vi "tm484_DSP.vi"() -> ()   [LabVIEW 2011]
panel:
  in  "SC Enable":bool
  in  "BG Enable":bool
  in  "Frame Averaging":i32(ring)=1 items=["1 Frame"=1, "2 Frames"=2, "4 Frames"=4]
  in  "Recursive Frames":i32(ring)=1 items=["1 Frame"=1, "2 Frames"=2, "4 Frames"=4, "8 Frames"=8, "16 Frames"=16]
  out "Image":u16[][](graph)
  in  "Quit":bool
  out "Error Out":errorcluster {"code" format="%.0x"}
  # "This is an example how to use the DSP functions.\nNot all camera have the DSP functions. Please\ncheck your camera manual to see your camera's\ncapabilities."
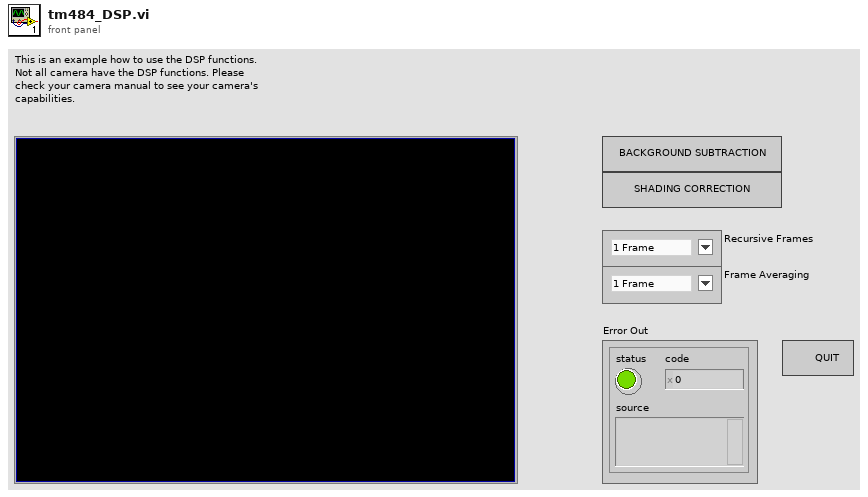
[diagram p1: front panel]
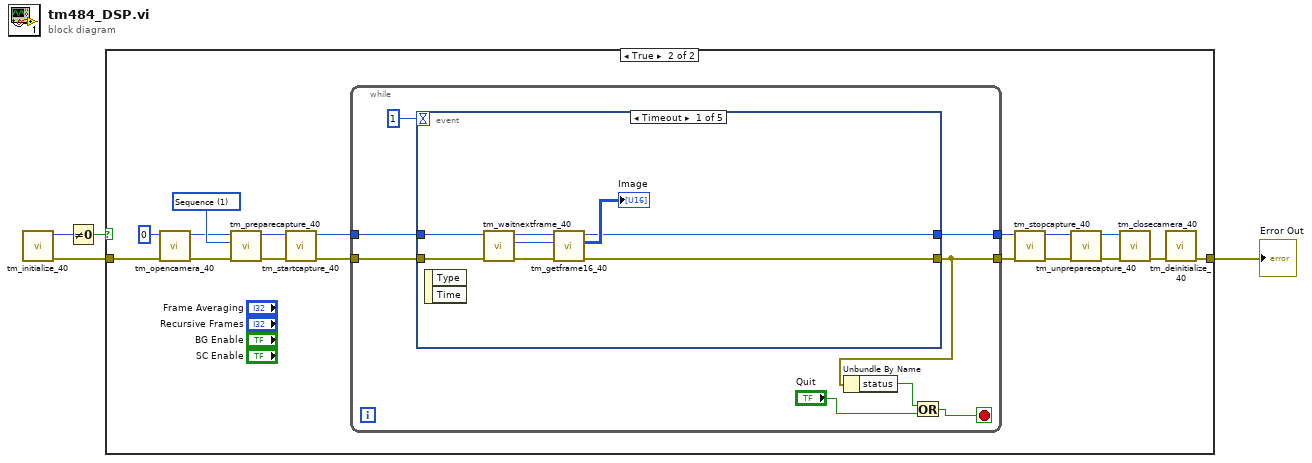
[diagram p0: block diagram]
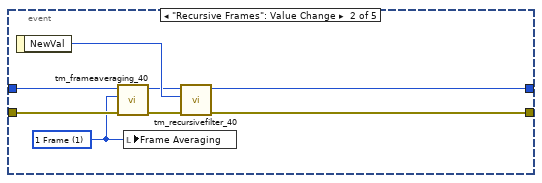
[diagram p3: hidden frame]
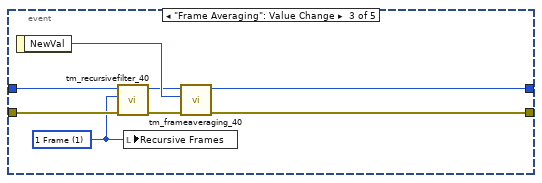
[diagram p4: hidden frame]
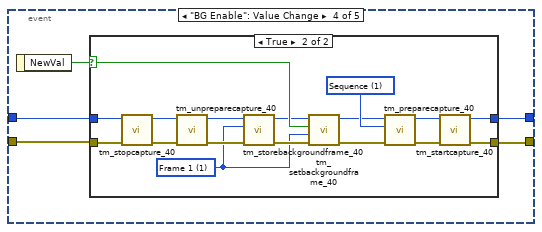
[diagram p5: hidden frame]
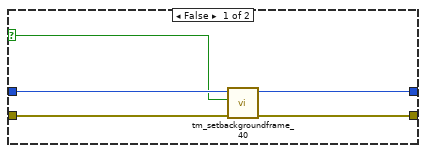
[diagram p6: hidden frame]
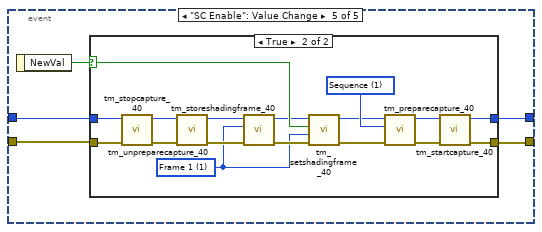
[diagram p7: hidden frame]
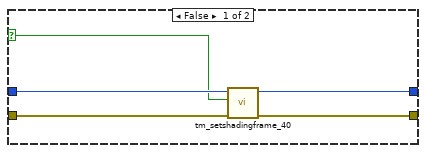
[diagram p8: hidden frame]
diagram:
  n1 = call <userlib>:"tm_initialize_40.vi"() -> ("error out"=w1:errorcluster, "Number Of Cameras"=w2:u32)  [unwired: 8 in, 2 out]
  n2 = Not Equal To 0?(x=w2) -> (x != 0?=w4:bool)
  n3 = case shown="True" w4 {
    tunnel: w1 -> [w5 w22]
    tunnel: [w5 w19] -> w3
    frame False {
    }
    frame True {
      w12 = 1 items=["Snap", "Sequence"] ("Capture mode")
      n4 = call <userlib>:"tm_opencamera_40.vi"("error in (no error)"=w22, "Camera Index"=u32 0) -> ("error out"=w9:errorcluster, "Handle out"=w8:u32)  [unwired: 7 in, 1 out]
      n5 = call <userlib>:"tm_preparecapture_40.vi"("error in (no error)"=w9, "Capture mode"=w12, "Handle in"=w8) -> ("error out"=w10:errorcluster, "Handle out"=w11:u32)  [unwired: 5 in, 2 out]
      n6 = call <userlib>:"tm_startcapture_40.vi"("error in (no error)"=w10, "Handle in"=w11) -> ("error out"=w6:errorcluster, "Handle out"=w7:u32)  [unwired: 8 in]
      n7 = while {
        tunnel: [w28] -> w15
        tunnel: [w24] -> w16
        tunnel: w7 -> [w30]
        tunnel: w6 -> [w29]
        stop <- w23 stop-if-true
        n8 = event shown="[0] Timeout" {
          selector: _ -> [_ _ _ _ _]
          dyn-events: _ -> [_ _ _ _ _]
          timeout: 1 -> [_ _ _ _ _]
          tunnel: w30 -> [w34 w42 w50 w58 w85]
          tunnel: w29 -> [w33 w43 w51 w57 w84]
          tunnel: [w31 w45 w53 w56 w83] -> w28
          tunnel: [w32 w44 w52 w55 w82] -> w24
          event Timeout {
            n9 = event-data() -> ()  [unwired: 1 in, 2 out]
            n10 = call <userlib>:"tm_waitnextframe_40.vi"("error in (no error)"=w33, "Handle in"=w34) -> ("error out"=w36:errorcluster, "Frame Index"=w38:i32, "Handle out"=w35:u32)  [unwired: 6 in, 1 out]
            n11 = call <userlib>:"tm_getframe16_40.vi"("error in (no error)"=w36, "Frame Index"=w38, "Handle in"=w35) -> ("error out"=w32:errorcluster, "Data"=→"Image":u16[][], "Handle out"=w31:u32)  [unwired: 5 in, 1 out]
          }
          event "Recursive Frames": Value Change {
            w39 = 1 items=["1 Frame"=1, "2 Frames"=2, "4 Frames"=4, "8 Frames"=8, "16 Frames"=16] ("Frames")
            n12 = event-data() -> ("NewVal"=w46:i32)  [unwired: 1 in]
            n13 = call <userlib>:"tm_frameaveraging_40.vi"("error in (no error)"=w43, "Frames"=w39, "Handle in"=w42) -> ("error out"=w40:errorcluster, "Handle out"=w41:u32)  [unwired: 7 in]
            n14 = local write "Frame Averaging"(w39) -> ()
            n15 = call <userlib>:"tm_recursivefilter_40.vi"("error in (no error)"=w40, "Frames"=w46, "Handle in"=w41) -> ("error out"=w44:errorcluster, "Handle out"=w45:u32)  [unwired: 7 in]
          }
          event "Frame Averaging": Value Change {
            w47 = 1 items=["1 Frame"=1, "2 Frames"=2, "4 Frames"=4, "8 Frames"=8, "16 Frames"=16] ("Frames")
            n16 = event-data() -> ("NewVal"=w54:i32)  [unwired: 1 in]
            n17 = call <userlib>:"tm_recursivefilter_40.vi"("error in (no error)"=w51, "Frames"=w47, "Handle in"=w50) -> ("error out"=w48:errorcluster, "Handle out"=w49:u32)  [unwired: 7 in]
            n18 = local write "Recursive Frames"(w47) -> ()
            n19 = call <userlib>:"tm_frameaveraging_40.vi"("error in (no error)"=w48, "Frames"=w54, "Handle in"=w49) -> ("error out"=w52:errorcluster, "Handle out"=w53:u32)  [unwired: 7 in]
          }
          event "BG Enable": Value Change {
            n20 = event-data() -> ("NewVal"=w59:bool)  [unwired: 1 in]
            n21 = case shown="True" w59 {
              selector: w59 -> [w60 w75]
              tunnel: w58 -> [w64 w78]
              tunnel: w57 -> [w63 w79]
              tunnel: [w62 w66] -> w56
              tunnel: [w61 w65] -> w55
              frame False {
                n22 = call <userlib>:"tm_setbackgroundframe_40.vi"("error in (no error)"=w63, "Enable"=w60, "Handle in"=w64) -> ("error out"=w61:errorcluster, "Handle out"=w62:u32)  [unwired: 7 in]
              }
              frame True {
                w69 = 1 items=["Snap", "Sequence"] ("Capture mode")
                w72 = 1 items=["Frame 1"=1, "Frame 2"=2, "Frame 3"=3, "Frame 4"=4] ("Frame")
                n23 = call <userlib>:"tm_stopcapture_40.vi"("error in (no error)"=w79, "Handle in"=w78) -> ("error out"=w81:errorcluster, "Handle out"=w80:u32)  [unwired: 8 in]
                n24 = call <userlib>:"tm_unpreparecapture_40.vi"("error in (no error)"=w81, "Handle in"=w80) -> ("error out"=w76:errorcluster, "Handle out"=w77:u32)  [unwired: 8 in]
                n25 = call <userlib>:"tm_storebackgroundframe_40.vi"("error in (no error)"=w76, "Frame"=w72, "Handle in"=w77) -> ("error out"=w73:errorcluster, "Handle out"=w74:u32)  [unwired: 7 in]
                n26 = call <userlib>:"tm_setbackgroundframe_40.vi"("error in (no error)"=w73, "Frame"=w72, "Enable"=w75, "Handle in"=w74) -> ("error out"=w68:errorcluster, "Handle out"=w67:u32)  [unwired: 6 in]
                n27 = call <userlib>:"tm_preparecapture_40.vi"("error in (no error)"=w68, "Capture mode"=w69, "Handle in"=w67) -> ("error out"=w71:errorcluster, "Handle out"=w70:u32)  [unwired: 5 in, 2 out]
                n28 = call <userlib>:"tm_startcapture_40.vi"("error in (no error)"=w71, "Handle in"=w70) -> ("error out"=w65:errorcluster, "Handle out"=w66:u32)  [unwired: 8 in]
              }
            }
          }
          event "SC Enable": Value Change {
            n29 = event-data() -> ("NewVal"=w86:bool)  [unwired: 1 in]
            n30 = case shown="True" w86 {
              selector: w86 -> [w87 w99]
              tunnel: w85 -> [w91 w105]
              tunnel: w84 -> [w90 w106]
              tunnel: [w89 w101] -> w83
              tunnel: [w88 w100] -> w82
              frame False {
                n31 = call <userlib>:"tm_setshadingframe_40.vi"("error in (no error)"=w90, "Enable"=w87, "Handle in"=w91) -> ("error out"=w88:errorcluster, "Handle out"=w89:u32)  [unwired: 7 in]
              }
              frame True {
                w102 = 1 items=["Snap", "Sequence"] ("Capture mode")
                w92 = 1 items=["Frame 1"=1, "Frame 2"=2, "Frame 3"=3, "Frame 4"=4] ("Frame")
                n32 = call <userlib>:"tm_stopcapture_40.vi"("error in (no error)"=w106, "Handle in"=w105) -> ("error out"=w108:errorcluster, "Handle out"=w107:u32)  [unwired: 8 in]
                n33 = call <userlib>:"tm_unpreparecapture_40.vi"("error in (no error)"=w108, "Handle in"=w107) -> ("error out"=w93:errorcluster, "Handle out"=w96:u32)  [unwired: 8 in]
                n34 = call <userlib>:"tm_storeshadingframe_40.vi"("error in (no error)"=w93, "Frame"=w92, "Handle in"=w96) -> ("error out"=w94:errorcluster, "Handle out"=w95:u32)  [unwired: 7 in]
                n35 = call <userlib>:"tm_setshadingframe_40.vi"("error in (no error)"=w94, "Frame"=w92, "Enable"=w99, "Handle in"=w95) -> ("error out"=w97:errorcluster, "Handle out"=w98:u32)  [unwired: 6 in]
                n36 = call <userlib>:"tm_preparecapture_40.vi"("error in (no error)"=w97, "Capture mode"=w102, "Handle in"=w98) -> ("error out"=w104:errorcluster, "Handle out"=w103:u32)  [unwired: 5 in, 2 out]
                n37 = call <userlib>:"tm_startcapture_40.vi"("error in (no error)"=w104, "Handle in"=w103) -> ("error out"=w100:errorcluster, "Handle out"=w101:u32)  [unwired: 8 in]
              }
            }
          }
        }
        n38 = Unbundle By Name(w24) -> ("status"=w27:bool)
        n39 = Or(x=w27, y="Quit") -> (x .or. y?=w23:bool)
      }
      n40 = call <userlib>:"tm_stopcapture_40.vi"("error in (no error)"=w16, "Handle in"=w15) -> ("error out"=w13:errorcluster, "Handle out"=w14:u32)  [unwired: 8 in]
      n41 = call <userlib>:"tm_unpreparecapture_40.vi"("error in (no error)"=w13, "Handle in"=w14) -> ("error out"=w18:errorcluster, "Handle out"=w17:u32)  [unwired: 8 in]
      n42 = call <userlib>:"tm_closecamera_40.vi"("error in (no error)"=w18, "Handle in"=w17) -> ("error out"=w20:errorcluster)  [unwired: 9 in]
      n43 = call <userlib>:"tm_deinitialize_40.vi"("error in (no error)"=w20) -> ("error out"=w19:errorcluster)  [unwired: 10 in]
    }
  }
  "Error Out" <- w3
